vi "Receive and Sort new Message.vi"(8 "error in":errorcluster, 10 "Data":variant, 11 "Message Log in":refnum<class "Message Log.lvclass">) -> (0 "error out":errorcluster, 3 "Message Log out":refnum<class "Message Log.lvclass">)   [LabVIEW 2017, in "Message Log.lvclass"]
uses:
  Message Log.lvclass
  Message Log.lvclass/Message Log.ctl
  <vilib>/addons/_Workers/Library/Classes/Worker/Debug Message Data.ctl
  <vilib>/addons/_Workers/Library/Classes/Message/Message Time Stamp.ctl
  <vilib>/addons/_Workers/Library/Case Label.ctl
  <vilib>/addons/_Workers/Library/Classes/Message/Priority (ALL).ctl
  <vilib>/addons/_Workers/Library/WID to Alias.vi
  <vilib>/addons/_Workers/Library/Classes/Message/Message.lvclass
  <vilib>/addons/_Workers/Library/Classes/Worker/Worker.lvclass
  <vilib>/addons/_Workers/Library/Workers.lvlib
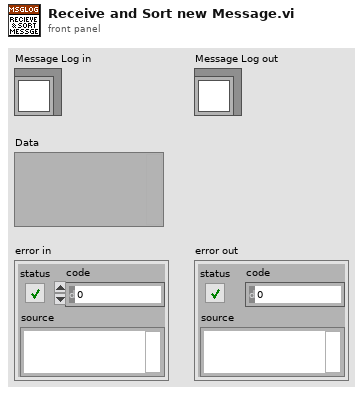
[diagram p1: front panel]
types:
  T1 = typedef "Workers.lvlib/Worker.lvclass/Debug Message Data.ctl" = cluster{"Time Stamp":T2, "Sender WID":string, "Sender Case":T3, "Recipient WID":string, "Recipient Case":T3, "Priority":T4, "Message String":string}
  T2 = typedef "Workers.lvlib/Message.lvclass/Message Time Stamp.ctl" = cluster{"Hi-Res Time (sec)":dbl, "Time":timestamp}
  T3 = typedef "Workers.lvlib/Case Label.ctl" = string
  T4 = typedef "Workers.lvlib/Message.lvclass/Priority (ALL).ctl" = enum16{"Low", "Normal", "High", "Critical"}
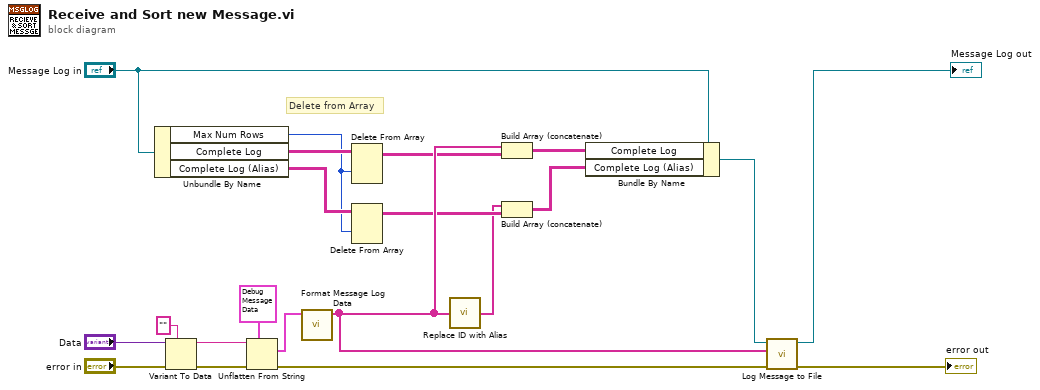
[diagram p0: block diagram]
diagram:
  # "Delete from Array"
  n1 = Unbundle By Name("Message Log in") -> ("Max Num Rows"=w2:i32, "Complete Log"=w3:string[][], "Complete Log (Alias)"=w6:string[][])
  n2 = Variant To Data(error in="error in", type="", Variant="Data") -> (data=w18:string, error out=w19:errorcluster)
  n3 = Unflatten From String(type=T1 {"Time Stamp"={"Hi-Res Time (sec)"=0.0, "Time"=timestamp(0 s since 1904-01-01)}, "Sender WID"="", "Sender Case"="", "Recipient WID"="", "Recipient Case"="", "Priority"=enum."Normal", "Message String"=""} ("Message Data"), binary string=w18, error in (no error)=w19) -> (value=w15:T1, error out=w14:errorcluster)  [unwired: 2 in, 1 out]
  n4 = call "Format Message Log Data.vi"("Message Data"=w15) -> ("Array"=w10:string[])  [unwired: 10 in]
  n5 = Delete From Array(array=w3, index (row)=w2) -> (array with subset deleted=w4:string[][])  [unwired: 2 in, 1 out]
  n6 = Delete From Array(array=w6, index (row)=w2) -> (array with subset deleted=w7:string[][])  [unwired: 2 in, 1 out]
  n7 = call "Replace ID with Alias.vi"("Message Log Data"=w10) -> ("Message Log Data (Short IDs)"=w1:string[])
  n8 = Build Array (concatenate)(w10, w4) -> (w5:string[][])
  n9 = Build Array (concatenate)(w1, w7) -> (w8:string[][])
  n10 = Bundle By Name(cluster="Message Log in", "Complete Log"=w5, "Complete Log (Alias)"=w8) -> (w11:refnum<class "Message Log.lvclass">)
  n11 = call "Log Message to File.vi"("error in (no error)"=w14, "Message Data"=w10, "Message Log in"=w11) -> ("error out"=→"error out":errorcluster, "Message Log out"=→"Message Log out":refnum<class "Message Log.lvclass">)  [unwired: 7 in]
